vi "SUB_FindExpanTime.vi"(2 "test item name":string, 3 "Input Source":string) -> (0 "expand_time":string)   [LabVIEW 2011]
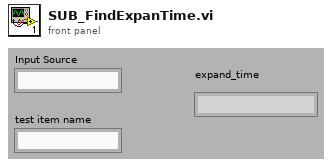
[diagram p1: front panel]
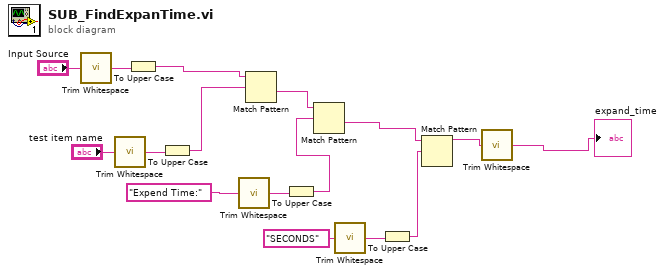
[diagram p0: block diagram]
diagram:
  n1 = call <vilib>:"Trim Whitespace.vi"("string"="Input Source") -> ("trimmed string"=w11:string)  [unwired: 1 in]
  n2 = call <vilib>:"Trim Whitespace.vi"("string"="test item name") -> ("trimmed string"=w16:string)  [unwired: 1 in]
  n3 = To Upper Case(1:w11) -> (0:w10:string)
  n4 = To Upper Case(1:w16) -> (0:w15:string)
  n5 = call <vilib>:"Trim Whitespace.vi"("string"="Expend Time:") -> ("trimmed string"=w14:string)  [unwired: 1 in]
  n6 = Match Pattern(string=w10, regular expression=w15) -> (after substring=w7:string)  [unwired: 1 in, 3 out]
  n7 = To Upper Case(1:w14) -> (0:w12:string)
  n8 = Match Pattern(string=w7, regular expression=w12) -> (after substring=w6:string)  [unwired: 1 in, 3 out]
  n9 = call <vilib>:"Trim Whitespace.vi"("string"="SECONDS") -> ("trimmed string"=w5:string)  [unwired: 1 in]
  n10 = To Upper Case(1:w5) -> (0:w4:string)
  n11 = Match Pattern(string=w6, regular expression=w4) -> (before substring=w2:string)  [unwired: 1 in, 3 out]
  n12 = call <vilib>:"Trim Whitespace.vi"("string"=w2) -> ("trimmed string"=→"expand_time":string)  [unwired: 1 in]
